vi "PKG_IMC_GetErrorReg.vi"(9 "axisnum":i32, 10 "err":u16[](array[numeric])=array[4097 elements], 11 "Handle":u32) -> (1 "function return":i32, 2 "err out":u16[](array[numeric]), 3 "Handle out":u32)   [LabVIEW 2018, in "IMC_Pkg4xxx.lvlib"]
doc: "PKG_IMC_GetErrorReg(IMC_HANDLE Handle, unsigned short err[], int axisnum);"
uses:
  IMC_Pkg4xxx.lvlib
  IMC_Pkg4xxx.dll
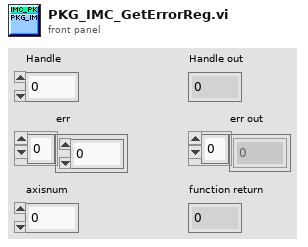
[diagram p1: front panel]
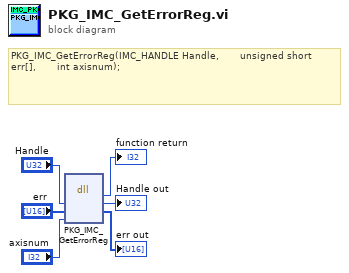
[diagram p0: block diagram]
diagram:
  # "PKG_IMC_GetErrorReg(IMC_HANDLE Handle, \t \t\t\t\tunsigned short err[], \t\t\t\t\t\tint axisnum);"
  n1 = dll-call lib="PTH2\\abs D做的项目航天测量驱动电机IMCAppincLabview32\nIMC_Pkg4xxx.*" fn="PKG_IMC_GetErrorReg"("Handle"="Handle", "err"="err", "axisnum"="axisnum") -> (→"function return":i32, "Handle"=→"Handle out":u32, "err"=→"err out":u16[])  [unwired: 4 in, 2 out]
